vi "AMC e.bloxx Read.vi"(8 "error in (no error)":errorcluster, 11 "VISA Resource Name":refnum<visa-resource-name>) -> (0 "error out":errorcluster, 2 "Module Response":string, 3 "VISA Resource Name out":refnum<visa-resource-name>)   [LabVIEW 2016]
doc: "<B>AMC - Analytik & Messtechnik GmbH Chemnitz</B>\n\nLabVIEW Drivers for e.bloxx series from Gantner Instruments\n\nThis VI is a driver subroutine and should not be used in an application. It reads char wise data from the serial interface specified in <B>VISA Resource Name</B>. The chars are assembled to a string which will be forwarded in <B>Module Response</B>. The VI stops reading data when either an end transmission control char arrived or an error occured while reading."
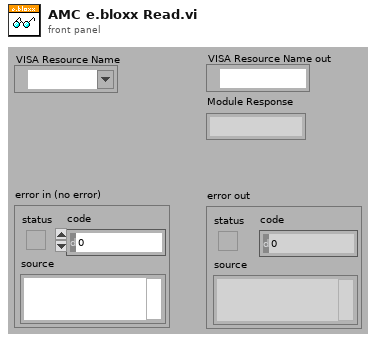
[diagram p1: front panel]
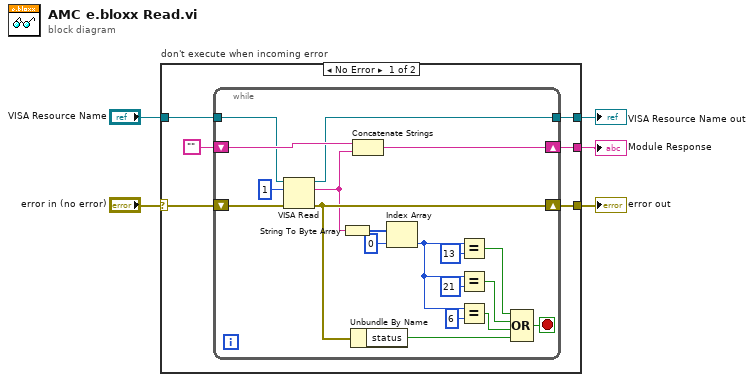
[diagram p0: block diagram]
diagram:
  n1 = case "don't execute when incoming error" shown="No Error" "error in (no error)" {
    selector: "error in (no error)" -> [w11 w32]
    tunnel: [w10 w32] -> w4
    tunnel: "VISA Resource Name" -> [w9 w31]
    tunnel: [w6 w31] -> w2
    tunnel: [w7 _] -> w1
    frame No Error {
      n2 = while {
        shift-right: [w28] -> w10
        shift-left: w11 -> [w30]
        tunnel: w9 -> [w13]
        shift-right: [w23] -> w7
        shift-left: "" -> [w25]
        tunnel: [w12] -> w6
        stop <- w14 stop-if-true
        n3 = VISA Read(VISA resource name=w13, byte count=u32 1, error in (no error)=w30) -> (VISA resource name out=w12:refnum<visa-resource-name>, read buffer=w24:string, error out=w28:errorcluster)  [unwired: 1 out]
        n4 = String To Byte Array(string=w24) -> (unsigned byte array=w27:u8[])
        n5 = Unbundle By Name(w28) -> ("status"=w18:bool)
        n6 = Concatenate Strings(w25, w24) -> (w23:string)
        n7 = Index Array(array=w27, index=0) -> (element=w19:u8)
        n8 = Equal?(x=w19, y=u8 13) -> (x = y?=w15:bool)
        n9 = Equal?(x=w19, y=u8 21) -> (x = y?=w16:bool)
        n10 = Equal?(x=w19, y=u8 6) -> (x = y?=w17:bool)
        n11 = Compound Arithmetic op=OR(w15, w16, w17, w18) -> (w14:bool)
      }
    }
    frame Error {
    }
  }
  "error out" <- w4
  "VISA Resource Name out" <- w2
  "Module Response" <- w1
